vi "MMEMory.vi"(8 "Error in (no error)":errorcluster, 9 "Filename":string, 10 "What":enum16{"CATalog", "DATA"}(ring), 11 "VISA resource":refnum<visa-resource-name>) -> (0 "Error out":errorcluster, 2 "Response":string, 3 "Dup VISA resource":refnum<visa-resource-name>)   [LabVIEW 2010]
doc: "Copyright (c) 2012 Metrolab Technology SA, Plan-les-Ouates, Geneva, Switzerland\nRead the THM1176 FLASH memory."
panel:
  # "MMEMory"
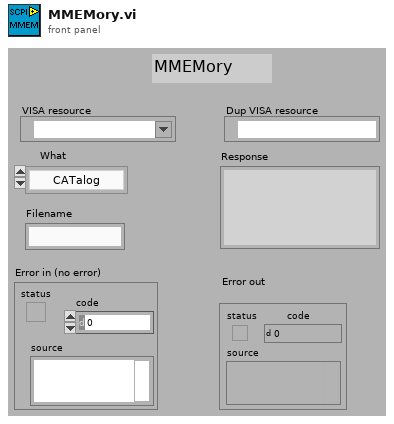
[diagram p1: front panel]
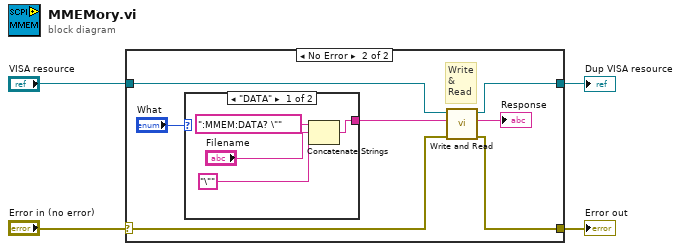
[diagram p0: block diagram]
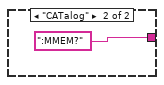
[diagram p3: hidden frame]
diagram:
  n1 = case shown="No Error" "Error in (no error)" {
    selector: "Error in (no error)" -> [w5 w10]
    tunnel: "VISA resource" -> [w6 w13]
    tunnel: [w6 w9] -> w1
    tunnel: [w5 w8] -> w4
    frame Error {
    }
    frame No Error {
      # "Write\n&\nRead"
      n2 = case shown="\"DATA\"" "What" {
        tunnel: [w17 ":MMEM?"] -> w7
        frame "DATA" {
          n3 = Concatenate Strings(":MMEM:DATA? \"" ("string"), "Filename", "\"" ("string")) -> (w17:string)
        }
        frame "CATalog" {
        }
      }
      n4 = call "Write and Read.vi"("Error in (no error)"=w10, "Command"=w7, "VISA resource"=w13) -> ("Error out"=w8:errorcluster, "Response"=→"Response":string, "Dup VISA resource"=w9:refnum<visa-resource-name>)  [unwired: 4 in, 2 out]
    }
  }
  "Error out" <- w4
  "Dup VISA resource" <- w1
